vi "Port.vi"(8 "error in (no error)":errorcluster, 11 "Node Ptr":T1 format="%.0x") -> (0 "error out":errorcluster)   [LabVIEW 2018, in "NI-XNET Monitor System Explorer.lvlib"]
uses:
  NI-XNET Monitor System Explorer.lvlib
  <vilib>/NI Veristand/Custom Device API/Custom Device Item Ref.ctl
  <vilib>/NI Veristand/Custom Device API/Get Item Property (I32).vi
  Shared/Constants.vi
  <vilib>/NI Veristand/Custom Device API/Get Item Property (String).vi
  <vilib>/NI Veristand/Custom Device API/Get Item Property (Boolean).vi
  <vilib>/NI Veristand/Custom Device API/Set Item Property (Boolean).vi
  <vilib>/NI Veristand/Custom Device API/Set Item Property (U32).vi
  <vilib>/NI Veristand/Custom Device API/Custom Device API.lvlib
  Shared/NI-XNET Monitor Shared.lvlib
  <vilib>/NI Veristand/Custom Device Tools/Custom Device Utility Library/Custom Device Utility Library.lvlib
panel:
  in  "Bus.Load.Period.ms":u32=1000 caption="Bus Load Measurement Period (ms)"
  in  "Disable Bus Load":bool caption="Disable Bus Load Measurement"
  out "Info Cluster":cluster{"String":string}={"String"="This port is disabled under the NI-XNET hardware configuration section. Go to the port definition to enable it."}
  in  "GoTo":bool
  in  "Force Disable Port Monitor":bool
  out "NI-XNET Port (SDF Path)":string
  out "Port Address":string
  in  "Header":cluster{"Section Name":string}={"Section Name"=" Port Settings"}
  in  "Description":string
  out "Port Name":string
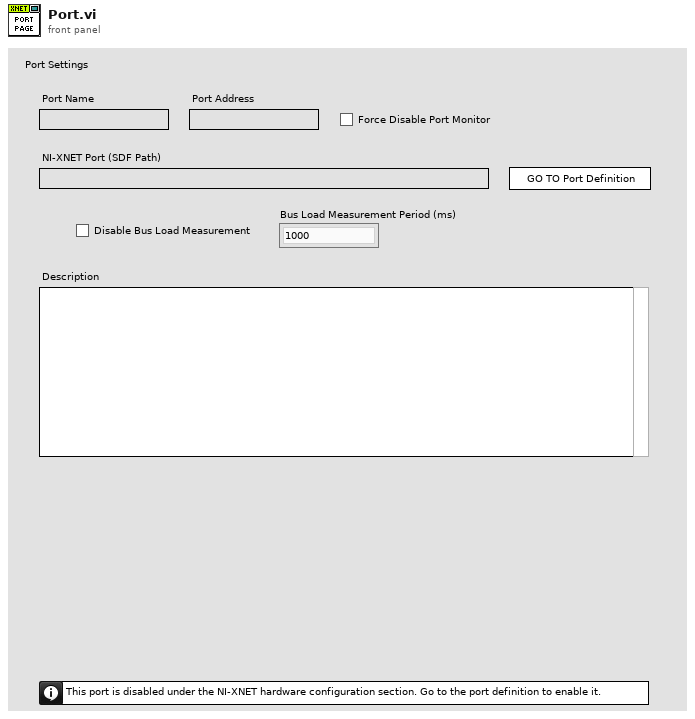
[diagram p1: front panel]
types:
  T1 = typedef "Custom Device API.lvlib/Custom Device Item Ref.ctl" = u64
  T2 = enum8{"Enabled", "Disabled", "Disabled and Grayed Out"}
  T3 = typedef "Custom Device API.lvlib/Custom Device Item Info.ctl" = cluster{"Name":string, "Is Channel":bool, "GUID":string, "Is Waveform":bool}
  T4 = typedef "NI-XNET Monitor Shared.lvlib/BusLoad.Settings.ctl" = cluster{"BusLoad.Disable":bool, "BusLoad.Periodms":u32}
  T5 = typedef "Custom Device API.lvlib/Custom Device Commands.ctl" = enum16{"Default", "Item renamed", "Shutdown", "Dynamic button pressed"}
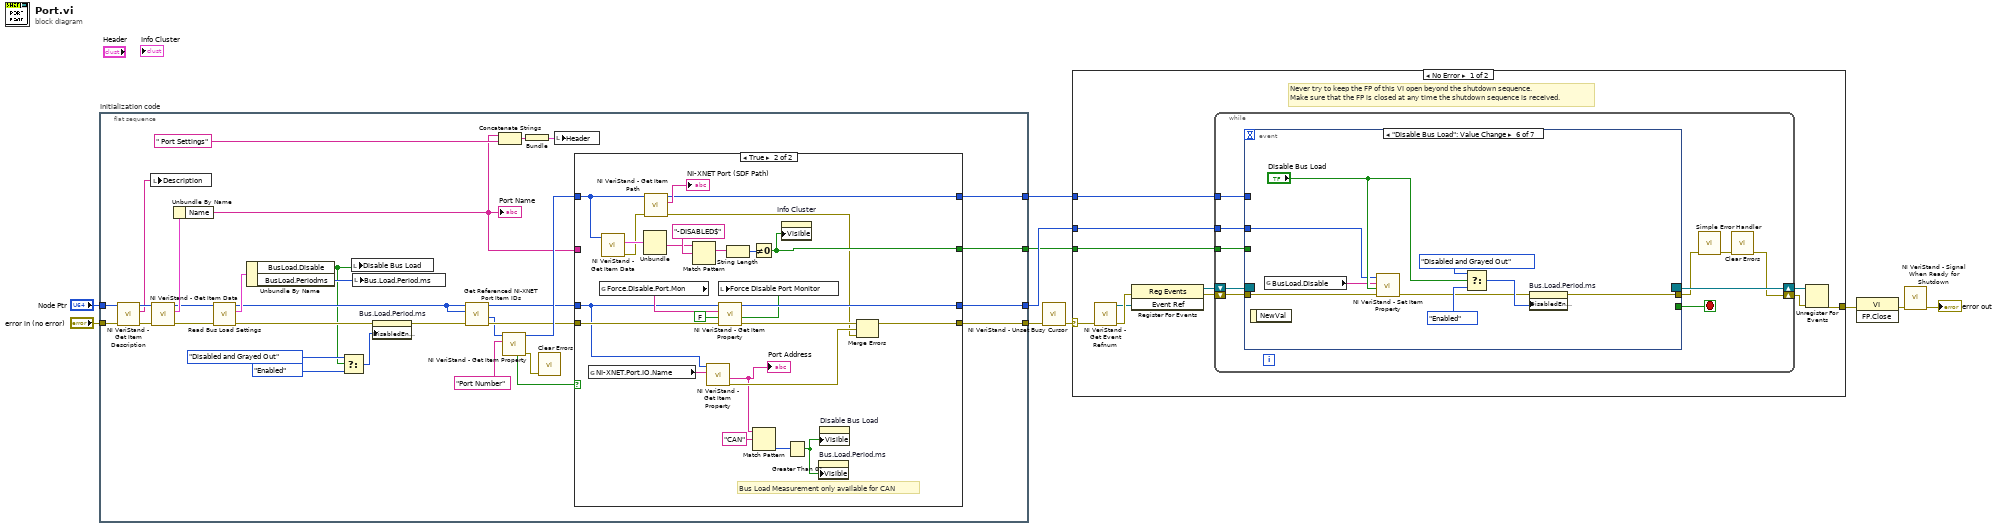
[diagram p0: block diagram]
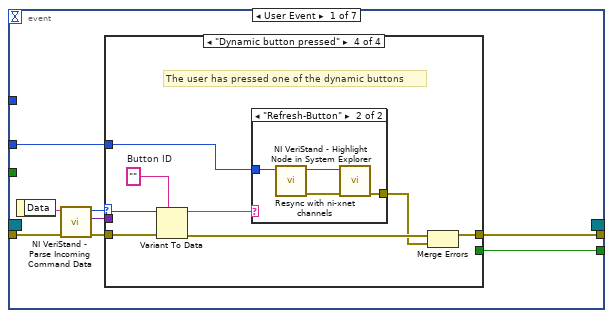
[diagram p2: hidden frame]
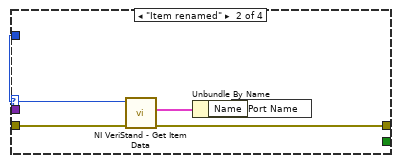
[diagram p4: hidden frame]
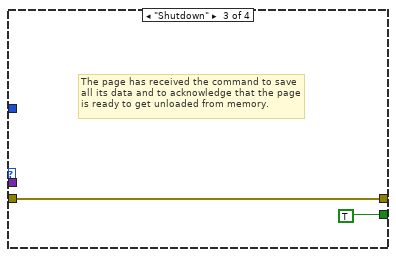
[diagram p5: hidden frame]
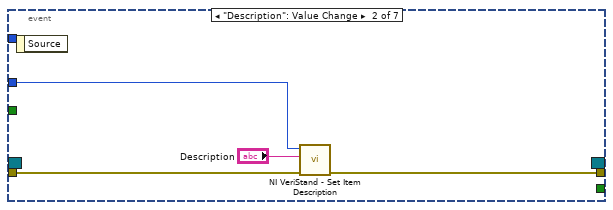
[diagram p7: hidden frame]
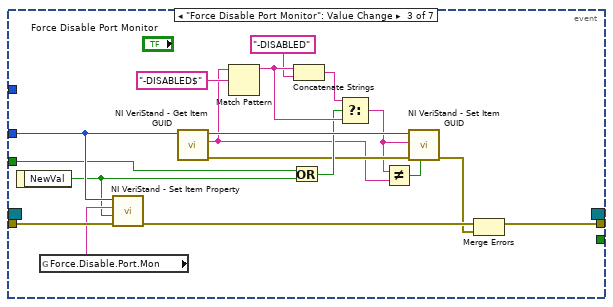
[diagram p8: hidden frame]
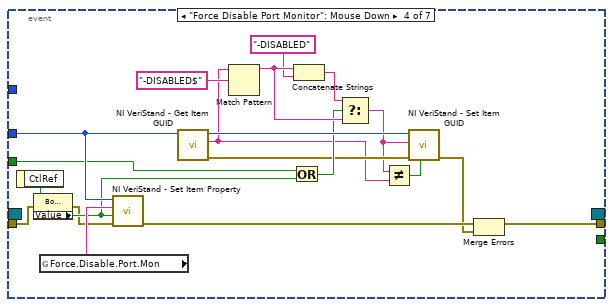
[diagram p9: hidden frame]
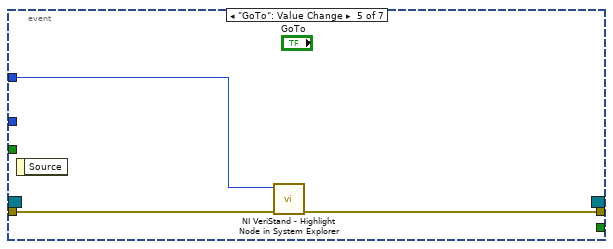
[diagram p10: hidden frame]
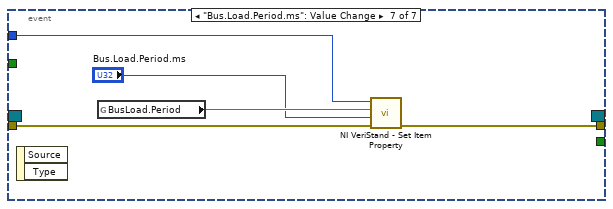
[diagram p11: hidden frame]
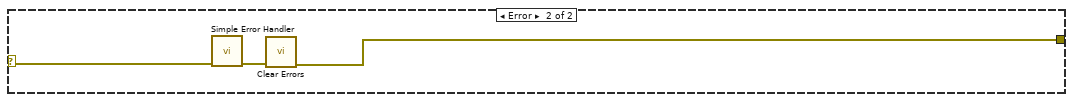
[diagram p12: hidden frame]
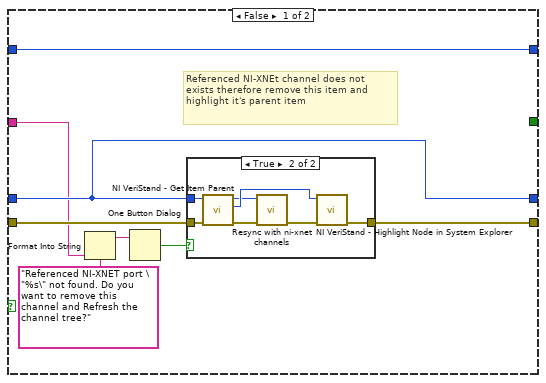
[diagram p13: hidden frame]
diagram:
  n1 = flat-sequence "Initialization code" {
    tunnel: "error in (no error)" -> [w41]
    tunnel: "Node Ptr" -> [w40]
    tunnel: [w34] -> w4
    tunnel: [w33] -> w3
    tunnel: [w35] -> w2
    tunnel: [w31] -> w1
    frame #0 {
      n2 = call <vilib>:"NI VeriStand - Get Item Description.vi"("error in (no error)"=w41, "Item Ref in"=w40) -> ("error out"=w38:errorcluster, "Description"=w39:string, "Item Ref out"=w42:T1)  [unwired: 7 out]
      n3 = local write "Description"(w39) -> ()
      n4 = call <vilib>:"NI VeriStand - Get Item Data.vi"("error in (no error)"=w38, "Item Ref in"=w42) -> ("error out"=w21:errorcluster, "Item Info"=w37:T3, "Item Ref out"=w20:T1)  [unwired: 7 out]
      n5 = Unbundle By Name(w37) -> ("Name"=w22:string)
      "Port Name" <- w22
      n6 = call "Read Bus Load Settings.vi"("error in (no error)"=w21, "Port Ref in"=w20) -> ("error out"=w15:errorcluster, "Bus Load Settings"=w19:T4, "Port Ref out"=w17:T1)  [unwired: 7 in]
      n7 = Unbundle By Name(w19) -> ("BusLoad.Disable"=w12:bool, "BusLoad.Periodms"=w18:u32)
      n8 = Select(t=T2."Disabled and Grayed Out" ("Disabled"), s=w12, f=T2."Enabled" ("Disabled")) -> (s? t:f=w11:T2)
      n9 = local write "Disable Bus Load"(w12) -> ()
      n10 = local write "Bus.Load.Period.ms"(w18) -> ()
      n11 = property on="Bus.Load.Period.ms" class="DigNum (strict)"(error in=w15, "DisabledEnum"=w11) -> (error out=w14:errorcluster)  [unwired: 1 in, 1 out]
      n12 = call "Get Referenced NI-XNET Port Item IDs.vi"("Error In"=w14, "CD Port Item Ref In"=w17, "Device Item Ref in in"=w17) -> ("Error Out"=w27:errorcluster, "NI-XNET Port Item Ref Out"=w26:T1, "Device Item Ref out"=w28:T1)  [unwired: 5 in, 1 out]
      n13 = Concatenate Strings(w22, " Port Settings" ("Section Name")) -> (w24:string)
      n14 = call-poly <vilib>:"NI VeriStand - Get Item Property.vi"("Property Name"="Port Number", "Item Ref in"=w26) -> ("error out"=w30:errorcluster, "Item Ref out"=w29:T1, "Found?"=w32:bool)  [unwired: 6 in, 1 out]
      n15 = Bundle(w24) -> (w25:cluster{string})  [unwired: 1 in]
      n16 = call <vilib>:"Clear Errors.vi"("error in (no error)"=w30) -> ()  [unwired: 5 in, 2 out]
      n17 = local write "Header"(w25) -> ()
      n18 = case shown="True" w32 {
        tunnel: w27 -> [w50 w68]
        tunnel: [w49 w67] -> w35
        tunnel: w28 -> [w47 w63]
        tunnel: [w47 w77] -> w34
        tunnel: [_ w74] -> w33
        tunnel: w29 -> [w48 w69]
        tunnel: [w48 w72] -> w31
        tunnel: w22 -> [w44 _]
        frame False {
          # "Referenced NI-XNEt channel does not exists therefore remove this item and highlight it's parent item"
          n19 = Format Into String(format string="Referenced NI-XNET port \"%s\" not found. Do you want to remove this channel and Refresh the channel tree?", w44) -> (resulting string=w45:string)  [unwired: 2 in, 1 out]
          n20 = One Button Dialog(message=w45) -> (true=w46:bool)  [unwired: 1 in]
          n21 = case shown="True" w46 {
            tunnel: w50 -> [w51 w58]
            tunnel: [w51 w57] -> w49
            tunnel: w47 -> [_ w56]
            frame False {
            }
            frame True {
              n22 = call <vilib>:"NI VeriStand - Get Item Parent.vi"("error in (no error)"=w58, "Item Ref in"=w56) -> ("error out"=w53:errorcluster, "Parent Ref"=w55:T1, "Item Ref out"=w54:T1)  [unwired: 6 in, 1 out]
              n23 = call "Resync with ni-xnet channels.vi"("Error In"=w53, "Device Item Ref in in"=w54) -> ("Error Out"=w52:errorcluster)  [unwired: 8 in, 1 out]
              n24 = call <vilib>:"NI VeriStand - Highlight Node in System Explorer.vi"("error in (no error)"=w52, "Item Ref in"=w55) -> ("error out"=w57:errorcluster)  [unwired: 8 in, 1 out]
            }
          }
        }
        frame True {
          # "Bus Load Measurement only available for CAN"
          n25 = global read "Constants.vi" "NI-XNET.Port.IO.Name"() -> (w71:string)
          n26 = global read "Constants.vi" "Force.Disable.Port.Mon"() -> (w78:string)
          n27 = call <vilib>:"NI VeriStand - Get Item Data.vi"("Item Ref in"=w69) -> ("error out"=w65:errorcluster, "Item Info"=w83:T3)  [unwired: 7 in, 2 out]
          n28 = Unbundle(w83) -> ("GUID"=w81:string)  [unwired: 3 out]
          n29 = call <vilib>:"NI VeriStand - Get Item Path.vi"("error in (no error)"=w65, "Item Ref in"=w69) -> ("error out"=w64:errorcluster, "Path"=→"NI-XNET Port (SDF Path)":string, "Item Ref out"=w72:T1)  [unwired: 6 in, 1 out]
          n30 = Match Pattern(string=w81, regular expression="-DISABLED$") -> (match substring=w80:string)  [unwired: 1 in, 3 out]
          n31 = call-poly <vilib>:"NI VeriStand - Get Item Property.vi"("Property Name"=w71, "Item Ref in"=w63) -> ("error out"=w70:errorcluster, "Value"=w62:string)  [unwired: 6 in, 2 out]
          "Port Address" <- w62
          n32 = call-poly <vilib>:"NI VeriStand - Get Item Property.vi"("error in (no error)"=w68, "Default Value"=FALSE, "Property Name"=w78, "Item Ref in"=w63) -> ("error out"=w66:errorcluster, "Value"=w75:bool, "Item Ref out"=w77:T1)  [unwired: 4 in, 1 out]
          n33 = local write "Force Disable Port Monitor"(w75) -> ()
          n34 = String Length(string=w80) -> (length=w79:i32)
          n35 = Not Equal To 0?(x=w79) -> (x != 0?=w74:bool)
          n36 = Match Pattern(string=w62, regular expression="CAN") -> (offset past match=w61:i32)  [unwired: 1 in, 3 out]
          n37 = property on="Info Cluster" class="Clust (strict)"("Visible"=w74) -> ()  [unwired: 2 in, 2 out]
          n38 = Greater Than 0?(x=w61) -> (x > 0?=w60:bool)
          n39 = property on="Bus.Load.Period.ms" class="DigNum (strict)"("Visible"=w60) -> ()  [unwired: 2 in, 2 out]
          n40 = property on="Disable Bus Load" class="Bool (strict)"("Visible"=w60) -> ()  [unwired: 2 in, 2 out]
          n41 = Merge Errors(w66, w70, w64) -> (w67:errorcluster)
        }
      }
    }
  }
  n42 = call <vilib>:"NI VeriStand - Unset Busy Cursor.vi"("error in (no error)"=w2) -> ("error out"=w6:errorcluster)  [unwired: 10 out]
  n43 = case shown="No Error" w6 {
    selector: w6 -> [w87 w194]
    tunnel: [w91 w192] -> w10
    tunnel: w4 -> [w85 _]
    tunnel: w3 -> [w86 _]
    tunnel: w1 -> [w84 _]
    frame No Error {
      # "Never try to keep the FP of this VI open beyond the shutdown sequence.\nMake sure that the FP is closed at any time the shutdown sequence is received."
      n44 = call <vilib>:"NI VeriStand - Get Event Refnum.vi"("error in (no error)"=w87) -> ("error out"=w94:errorcluster, "Event Ref"=w90:refnum<user-event>)  [unwired: 9 out]
      n45 = register-events(error in=w94, w90) -> (reference out=w88:refnum<event-registration>, error out=w89:errorcluster)  [unwired: 1 in]
      n46 = while {
        tunnel: w85 -> [w100]
        shift-right: [w97] -> w92
        shift-left: w89 -> [w103]
        shift-right: [w104] -> w93
        shift-left: w88 -> [w102]
        tunnel: w86 -> [w96]
        tunnel: w84 -> [w95]
        stop <- w101 stop-if-true
        n47 = event shown="[5] \"Disable Bus Load\": Value Change" {
          selector: w102 -> [_ _ _ _ _ _ _]
          dyn-events: [_ _ _ _ _ _ _] -> w104
          timeout: _ -> [_ _ _ _ _ _ _]
          tunnel: w103 -> [w112 w135 w154 w155 w176 w182 w189]
          tunnel: [w108 _ _ _ _ _ _] -> w101
          tunnel: [w107 w134 w147 w169 w175 w186 w190] -> w99
          tunnel: w100 -> [w106 w136 w151 w172 _ w178 w188]
          tunnel: w96 -> [_ _ w140 w162 _ _ _]
          tunnel: w95 -> [_ _ _ _ w177 _ _]
          event User Event {
            n48 = event-data() -> ("Data"=w111:string)  [unwired: 1 out]
            n49 = call <vilib>:"NI VeriStand - Parse Incoming Command Data.vi"("error in (no error)"=w112, "Incoming data"=w111) -> ("error out"=w110:errorcluster, "Outgoing data"=w105:variant, "Action"=w109:T5)  [unwired: 7 out]
            n50 = case shown="\"Dynamic button pressed\"" w109 {
              tunnel: w110 -> [w113 w118 w119 w128]
              tunnel: [_ _ TRUE _] -> w108
              tunnel: [w113 w115 w119 w122] -> w107
              tunnel: w106 -> [_ w117 _ w123]
              tunnel: w105 -> [_ _ _ w127]
              frame "Default", Default {
              }
              frame "Item renamed" {
                n51 = call <vilib>:"NI VeriStand - Get Item Data.vi"("error in (no error)"=w118, "Item Ref in"=w117) -> ("error out"=w115:errorcluster, "Item Info"=w116:T3)  [unwired: 8 out]
                n52 = Unbundle By Name(w116) -> ("Name"=w114:string)
                n53 = local write "Port Name"(w114) -> ()
              }
              frame "Shutdown" {
                # "The page has received the command to save all its data and to acknowledge that the page is ready to get unloaded from memory."
              }
              frame "Dynamic button pressed" {
                w126 = ""  # Button ID
                # "The user has pressed one of the dynamic buttons"
                n54 = Variant To Data(error in=w128, type=w126, Variant=w127) -> (data=w124:string, error out=w125:errorcluster)
                n55 = case shown="\"Refresh-Button\"" w124 {
                  tunnel: w123 -> [_ w132]
                  tunnel: [_ w129] -> w121
                  frame Default {
                  }
                  frame "Refresh-Button" {
                    n56 = call "Resync with ni-xnet channels.vi"("Device Item Ref in in"=w132) -> ("Error Out"=w130:errorcluster, "Device Item Ref out"=w131:T1)  [unwired: 9 in]
                    n57 = call <vilib>:"NI VeriStand - Highlight Node in System Explorer.vi"("error in (no error)"=w130, "Item Ref in"=w131) -> ("error out"=w129:errorcluster)  [unwired: 8 in, 1 out]
                  }
                }
                n58 = Merge Errors(w125, w121) -> (w122:errorcluster)
              }
            }
          }
          event "Description": Value Change {
            n59 = event-data() -> ()  [unwired: 2 out]
            n60 = call <vilib>:"NI VeriStand - Set Item Description.vi"("error in (no error)"=w135, "Description"="Description", "Item Ref in"=w136) -> ("error out"=w134:errorcluster)  [unwired: 8 out]
          }
          event "Force Disable Port Monitor": Value Change {
            n61 = event-data() -> ("NewVal"=w148:bool)  [unwired: 1 out]
            n62 = global read "Constants.vi" "Force.Disable.Port.Mon"() -> (w152:string)
            n63 = call-poly <vilib>:"NI VeriStand - Set Item Property.vi"("error in (no error)"=w154, "Value"=w148, "Property Name"=w152, "Item Ref in"=w151) -> ("error out"=w153:errorcluster)  [unwired: 5 in, 2 out]
            n64 = call <vilib>:"NI VeriStand - Get Item GUID.vi"("Item Ref in"=w151) -> ("error out"=w141:errorcluster, "GUID"=w137:string, "Item Ref out"=w150:T1)  [unwired: 8 in]
            n65 = Match Pattern(string=w137, regular expression="-DISABLED$") -> (before substring=w144:string)  [unwired: 1 in, 3 out]
            n66 = Or(x=w140, y=w148) -> (x .or. y?=w142:bool)
            n67 = Concatenate Strings(w144, "-DISABLED" ("regular expression")) -> (w145:string)
            n68 = Select(t=w145, s=w142, f=w144) -> (s? t:f=w138:string)
            n69 = Not Equal?(x=w138, y=w137) -> (x != y?=w139:bool)
            n70 = call <vilib>:"NI VeriStand - Set Item GUID.vi"("Refresh System Explorer Tree? (F)"=w139, "error in (no error)"=w141, "GUID"=w138, "Item Ref in"=w150) -> ("error out"=w146:errorcluster)  [unwired: 6 in, 1 out]
            n71 = Merge Errors(w153, w146) -> (w147:errorcluster)
          }
          event "Force Disable Port Monitor": Mouse Down {
            n72 = event-data() -> ("CtlRef"=w158:refnum<vi>)  [unwired: 1 out]
            n73 = property class="Bool (strict)"(reference=w158, error in=w155) -> (error out=w156:errorcluster, "Value"=w157:bool)  [unwired: 1 out]
            n74 = global read "Constants.vi" "Force.Disable.Port.Mon"() -> (w173:string)
            n75 = call-poly <vilib>:"NI VeriStand - Set Item Property.vi"("error in (no error)"=w156, "Value"=w157, "Property Name"=w173, "Item Ref in"=w172) -> ("error out"=w174:errorcluster)  [unwired: 5 in, 2 out]
            n76 = call <vilib>:"NI VeriStand - Get Item GUID.vi"("Item Ref in"=w172) -> ("error out"=w163:errorcluster, "GUID"=w159:string, "Item Ref out"=w171:T1)  [unwired: 8 in]
            n77 = Match Pattern(string=w159, regular expression="-DISABLED$") -> (before substring=w166:string)  [unwired: 1 in, 3 out]
            n78 = Or(x=w162, y=w157) -> (x .or. y?=w164:bool)
            n79 = Concatenate Strings(w166, "-DISABLED" ("regular expression")) -> (w167:string)
            n80 = Select(t=w167, s=w164, f=w166) -> (s? t:f=w160:string)
            n81 = Not Equal?(x=w160, y=w159) -> (x != y?=w161:bool)
            n82 = call <vilib>:"NI VeriStand - Set Item GUID.vi"("Refresh System Explorer Tree? (F)"=w161, "error in (no error)"=w163, "GUID"=w160, "Item Ref in"=w171) -> ("error out"=w168:errorcluster)  [unwired: 6 in, 1 out]
            n83 = Merge Errors(w174, w168) -> (w169:errorcluster)
          }
          event "GoTo": Value Change {
            n84 = event-data() -> ()  [unwired: 2 out]
            n85 = call <vilib>:"NI VeriStand - Highlight Node in System Explorer.vi"("error in (no error)"=w176, "Item Ref in"=w177) -> ("error out"=w175:errorcluster)  [unwired: 8 in, 1 out]
          }
          event "Disable Bus Load": Value Change {
            n86 = event-data() -> ()  [unwired: 2 out]
            n87 = global read "Constants.vi" "BusLoad.Disable"() -> (w179:string)
            n88 = call-poly <vilib>:"NI VeriStand - Set Item Property.vi"("error in (no error)"=w182, "Value"="Disable Bus Load", "Property Name"=w179, "Item Ref in"=w178) -> ("error out"=w181:errorcluster)  [unwired: 5 in, 2 out]
            n89 = Select(t=T2."Disabled and Grayed Out" ("Disabled"), s="Disable Bus Load", f=T2."Enabled" ("Disabled")) -> (s? t:f=w183:T2)
            n90 = property on="Bus.Load.Period.ms" class="DigNum (strict)"(error in=w181, "DisabledEnum"=w183) -> (error out=w186:errorcluster)  [unwired: 1 in, 1 out]
          }
          event "Bus.Load.Period.ms": Value Change {
            n91 = event-data() -> ()  [unwired: 3 out]
            n92 = global read "Constants.vi" "BusLoad.Period"() -> (w191:string)
            n93 = call-poly <vilib>:"NI VeriStand - Set Item Property.vi"("error in (no error)"=w189, "Value"="Bus.Load.Period.ms", "Property Name"=w191, "Item Ref in"=w188) -> ("error out"=w190:errorcluster)  [unwired: 5 in, 2 out]
          }
        }
        n94 = call <vilib>:"Simple Error Handler.vi"("error in (no error)"=w99) -> ("error out"=w98:errorcluster)  [unwired: 1 in, 7 out]
        n95 = call <vilib>:"Clear Errors.vi"("error in (no error)"=w98) -> ("error out"=w97:errorcluster)  [unwired: 1 in, 5 out]
      }
      n96 = Unregister For Events(event registration refnum=w93, error in=w92) -> (error out=w91:errorcluster)
    }
    frame Error {
      n97 = call <vilib>:"Simple Error Handler.vi"("error in (no error)"=w194) -> ("error out"=w193:errorcluster)  [unwired: 1 in, 7 out]
      n98 = call <vilib>:"Clear Errors.vi"("error in (no error)"=w193) -> ("error out"=w192:errorcluster)  [unwired: 1 in, 5 out]
    }
  }
  n99 = invoke class="VI" method="FP.Close"(error in=w10) -> (error out=w9:errorcluster)  [unwired: 2 in, 2 out]
  n100 = call <vilib>:"NI VeriStand - Signal When Ready for Shutdown.vi"("error in (no error)"=w9) -> ("error out"=→"error out":errorcluster)  [unwired: 10 out]
